vi "Create Error Log Text.vi"(2 "Module Init Timestamp":timestamp, 3 "Error_Log_Setting":T1, 4 "Error to be logged":T2) -> (0 "Number of characters":i32, 1 "Text to be written to error log file":string)   [LabVIEW 2016, in "Error Manager.lvlib" / "Error Log.lvclass"]
uses:
  Error Log.lvclass
  Error Manager.lvlib
  Error Type (enum).ctl
  Error to be logged (cluster).ctl
  Settings/Error_Log_Setting (enum).ctl
  Settings/Settings.lvclass
panel:
  # "Input\nInputs to the VI"
  # "Development\nControls or indicators that are useful for development or testing, but which are not outputs of the VI."
  # "Output\nOutputs of the VI"
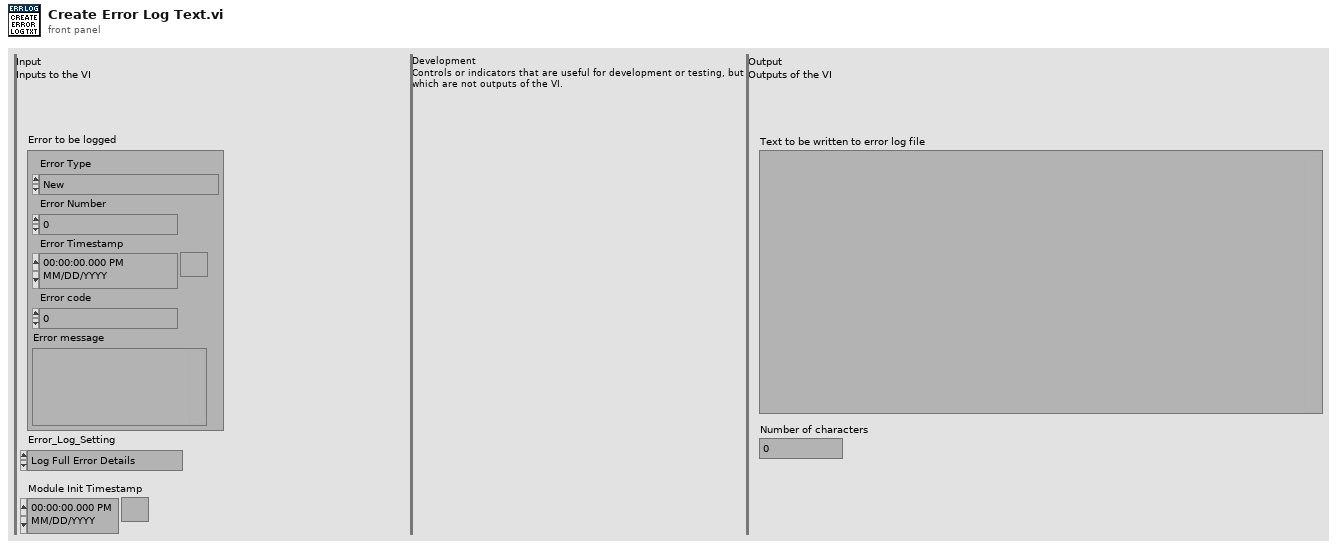
[diagram p1: front panel]
types:
  T1 = typedef "Error Manager.lvlib/Settings.lvclass/Error_Log_Setting (enum).ctl" = enum16{"Log Full Error Details", "Log Error Codes Only", "Do Not Log"}
  T2 = typedef "Error Manager.lvlib/Error Log.lvclass/Error to be logged (cluster).ctl" = cluster{"Error Type":T3, "Error Number":i32, "Error Timestamp":timestamp, "Error code":i32, "Error message":string}
  T3 = typedef "Error Manager.lvlib/Error Log.lvclass/Error Type (enum).ctl" = enum16{"New", "Identical to last logged error"}
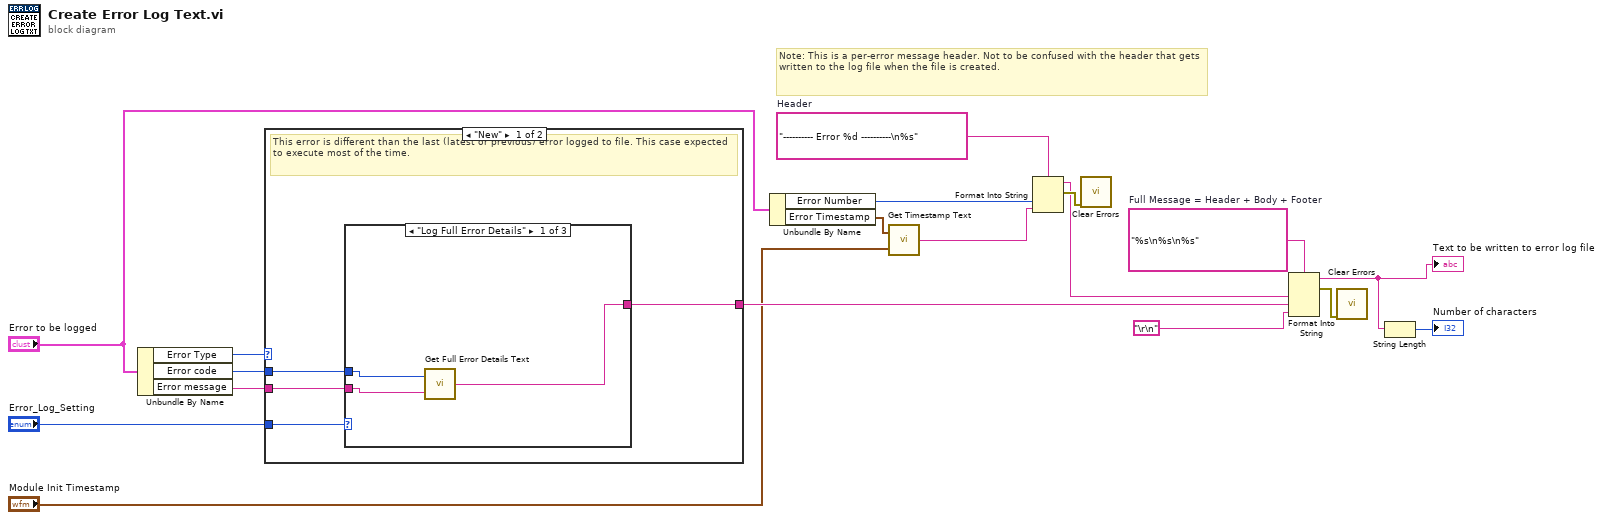
[diagram p0: block diagram]
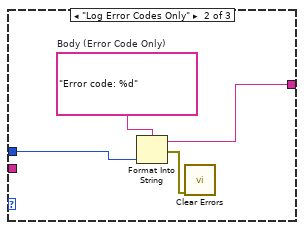
[diagram p2: hidden frame]
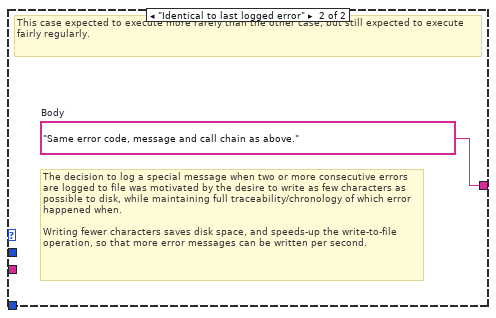
[diagram p4: hidden frame]
diagram:
  w11 = "%s\n%s\n%s"  # Full Message = Header + Body + Footer
  w15 = "---------- Error %d ----------\n%s"  # Header
  # "Note: This is a per-error message header. Not to be confused with the header that gets written to the log file when the file is created."
  n1 = Unbundle By Name("Error to be logged") -> ("Error Type"=w16:T3, "Error code"=w18:i32, "Error message"=w17:string)
  n2 = case shown="\"New\"" w16 {
    tunnel: [w22 w30] -> w9
    tunnel: w18 -> [w21 _]
    tunnel: w17 -> [w20 _]
    tunnel: "Error_Log_Setting" -> [w19 _]
    frame "New" {
      # "This error is different than the last (latest or previous) error logged to file. This case expected to execute most of the time."
      n3 = case shown="\"Log Full Error Details\"" w19 {
        tunnel: [w23 w28 _] -> w22
        tunnel: w21 -> [w25 w26 _]
        tunnel: w20 -> [w24 _ _]
        frame "Log Full Error Details" {
          n4 = call "Get Full Error Details Text.vi"("Error Message"=w24, "Error Code"=w25) -> ("Full Error Details Text"=w23:string)
        }
        frame "Log Error Codes Only" {
          w29 = "Error code: %d"  # Body (Error Code Only)
          n5 = Format Into String(format string=w29, w26) -> (resulting string=w28:string, error out=w27:errorcluster)  [unwired: 2 in]
          n6 = call <vilib>:"Clear Errors.vi"("error in (no error)"=w27) -> ()  [unwired: 5 in, 2 out]
        }
        frame "Do Not Log" {
          # "This case should never execute. This VI should execute only if the Error_Log_Setting is different than \"Do Not Log\"."
        }
      }
    }
    frame "Identical to last logged error" {
      w30 = "Same error code, message and call chain as above."  # Body
      # "The decision to log a special message when two or more consecutive errors are logged to file was motivated by the desire to write as few characters as possible to disk, while maintaining full traceability/chronology of which error happened when.\n\nWriting fewer characters saves disk space, and speeds-up the write-to-file operation, so that more error messages can be written per second."
      # "This case expected to execute more rarely than the other case, but still expected to execute fairly regularly."
    }
  }
  n7 = Unbundle By Name("Error to be logged") -> ("Error Number"=w13:i32, "Error Timestamp"=w2:timestamp)
  n8 = call "Get Timestamp Text.vi"("Module Init Timestamp"="Module Init Timestamp", "Error Timestamp"=w2) -> ("Timestamp String"=w3:string)
  n9 = Format Into String(format string=w15, w13, w3) -> (resulting string=w10:string, error out=w12:errorcluster)  [unwired: 2 in]
  n10 = call <vilib>:"Clear Errors.vi"("error in (no error)"=w12) -> ()  [unwired: 5 in, 2 out]
  n11 = Format Into String(format string=w11, w10, w9, "\r\n") -> (resulting string=w6:string, error out=w7:errorcluster)  [unwired: 2 in]
  "Text to be written to error log file" <- w6
  n12 = call <vilib>:"Clear Errors.vi"("error in (no error)"=w7) -> ()  [unwired: 5 in, 2 out]
  n13 = String Length(string=w6) -> (length=→"Number of characters":i32)
